vi "ReadOutTiffPicture.vi"(0 "Path":path=path "\\\\Walnuss\\Silverbrick/Lab/Stefan/Data/041108/C63/s_0001.b16", 1 "Binning size":i32) -> (2 "Indicator":dbl[][](array[numeric]), 3 "Width":i32, 4 "Height":i32)   [LabVIEW 2010]
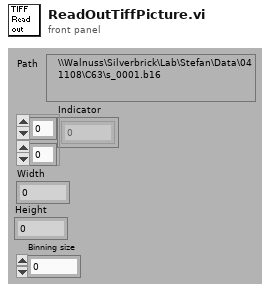
[diagram p1: front panel]
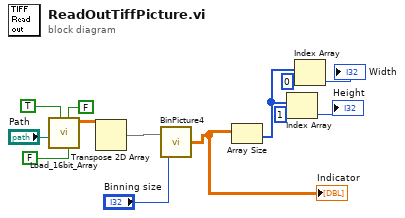
[diagram p0: block diagram]
diagram:
  n1 = call "Load_16bit_Array.vi"("Load in PCO Format"=FALSE, "Load Array"=FALSE, "Take Full Path"=TRUE, "Path"="Path") -> ("Fluorescence Image"=w12:dbl[][])  [unwired: 6 in, 1 out]
  n2 = Transpose 2D Array(2D array=w12) -> (transposed array=w3:dbl[][])
  n3 = call "BinPicture4.vi"("Binning size"="Binning size", "To bin"=w3) -> ("Output"=w2:dbl[][])
  "Indicator" <- w2
  n4 = Array Size(array=w2) -> (size(s)=w9:i32[])
  n5 = Index Array(array=w9, index=1) -> (element=→"Height":i32)
  n6 = Index Array(array=w9, index=0) -> (element=→"Width":i32)
